vi "Initialise.vi"(8 "error in (no error)":errorcluster, 11 "LINX-ADS1256 in":refnum<class "LINX-ADS1256.lvclass">) -> (0 "error out":errorcluster, 3 "LINX-ADS1256 out":refnum<class "LINX-ADS1256.lvclass">)   [LabVIEW 2020, in "LINX-ADS1256.lvclass"]
uses:
  LINX-ADS1256.lvclass
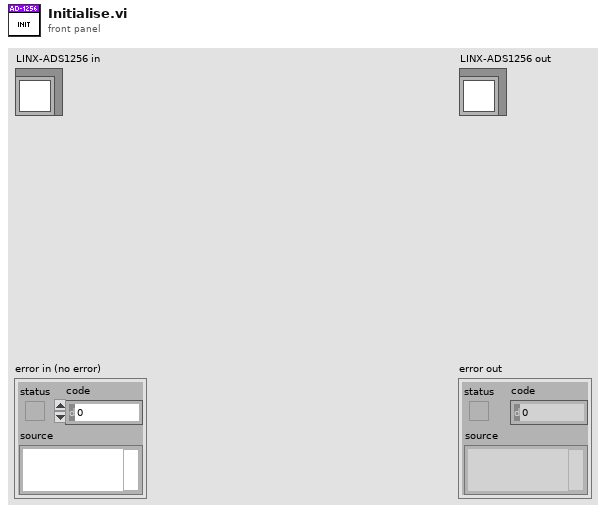
[diagram p1: front panel]
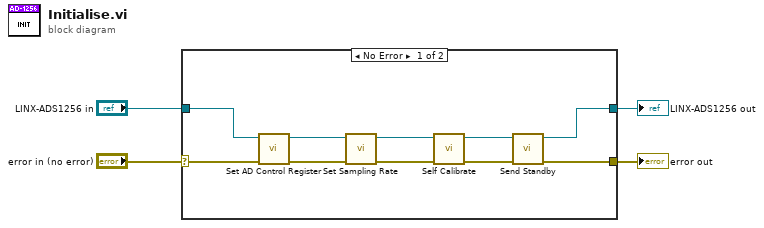
[diagram p0: block diagram]
diagram:
  n1 = case shown="No Error" "error in (no error)" {
    selector: "error in (no error)" -> [w11 w16]
    tunnel: [w5 w16] -> w3
    tunnel: [w6 w15] -> w1
    tunnel: "LINX-ADS1256 in" -> [w12 w15]
    frame No Error {
      n2 = call "Set AD Control Register.vi"("error in (no error)"=w11, "LINX-ADS1256 in"=w12) -> ("error out"=w10:errorcluster, "LINX-ADS1256 out"=w9:refnum<class "LINX-ADS1256.lvclass">)  [unwired: 8 in]
      n3 = call "Set Sampling Rate.vi"("error in (no error)"=w10, "LINX-ADS1256 in"=w9) -> ("error out"=w13:errorcluster, "LINX-ADS1256 out"=w14:refnum<class "LINX-ADS1256.lvclass">)  [unwired: 8 in]
      n4 = call "Self Calibrate.vi"("error in (no error)"=w13, "LINX-ADS1256 in"=w14) -> ("error out"=w7:errorcluster, "LINX-ADS1256 out"=w8:refnum<class "LINX-ADS1256.lvclass">)  [unwired: 8 in]
      n5 = call "Send Standby.vi"("error in (no error)"=w7, "LINX-ADS1256 in"=w8) -> ("error out"=w5:errorcluster, "LINX-ADS1256 out"=w6:refnum<class "LINX-ADS1256.lvclass">)  [unwired: 8 in]
    }
    frame Error {
    }
  }
  "error out" <- w3
  "LINX-ADS1256 out" <- w1
